vi "sendCmdFromTcpClientA.vi"(8 "error in (no error)":errorcluster, 11 "connectionID_A":refnum<k5>) -> (0 "error out":errorcluster, 2 "ack received":string[](array[string]), 3 "connectionID_A":refnum<k5>)   [LabVIEW 2018]
doc: "Generate commands as JSON packets and send them to TCP server, and then read the response from TCP server."
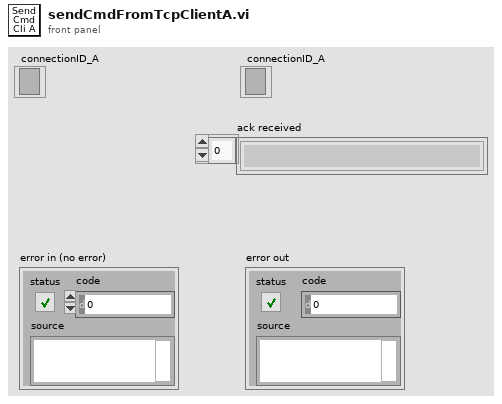
[diagram p1: front panel]
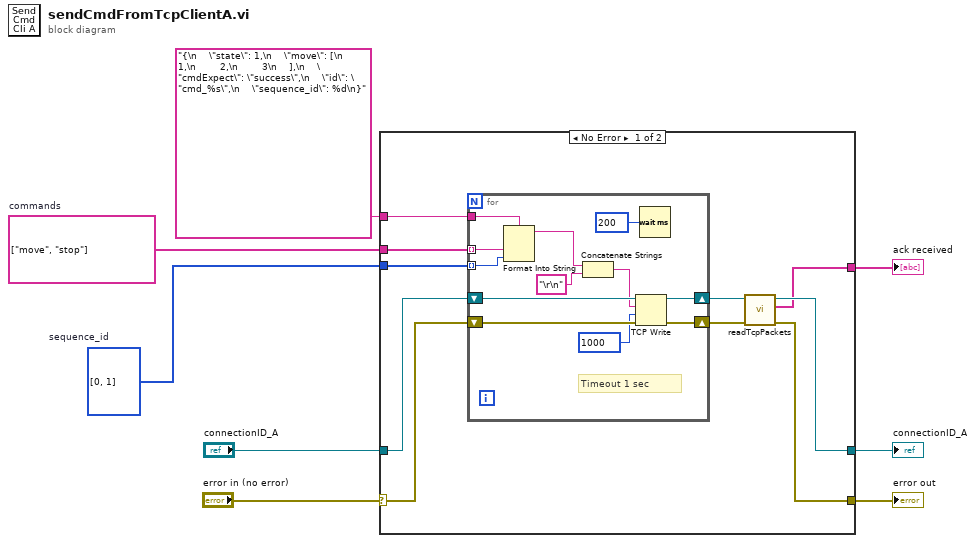
[diagram p0: block diagram]
diagram:
  w1 = i32[] [0, 1]  # sequence_id
  w2 = string[] ["move", "stop"]  # commands
  n1 = case shown="No Error" "error in (no error)" {
    selector: "error in (no error)" -> [w9 w32]
    tunnel: [w13 w31] -> w8
    tunnel: [w12 w32] -> w6
    tunnel: [w11 _] -> w5
    tunnel: "connectionID_A" -> [w18 w31]
    tunnel: "{\n    \"state\": 1,\n    \"move\": [\n        1,\n        2,\n        3\n    ],\n    \"cmdExpect\": \"success\",\n    \"id\": \"cmd_%s\",\n    \"sequence_id\": %d\n}" ("Display") -> [w10 _]
    tunnel: w2 -> [w17 _]
    tunnel: w1 -> [w16 _]
    frame No Error {
      n2 = for {
        shift-right: [w29] -> w14
        shift-left: w9 -> [w25]
        shift-right: [w27] -> w15
        shift-left: w18 -> [w26]
        tunnel: w10 -> [w23]
        tunnel: w17 -> [w22] mode=indexing
        tunnel: w16 -> [w21] mode=indexing
        # "Timeout 1 sec"
        n3 = Format Into String(format string=w23, w22, w21) -> (resulting string=w20:string)  [unwired: 2 in, 1 out]
        n4 = Concatenate Strings(w20, "\r\n" ("string")) -> (w24:string)
        n5 = TCP Write(connection ID=w26, data in=w24, error in (no error)=w25, 9:1000 ("timeout ms (25000)")) -> (connection ID out=w27:refnum<k5>, error out=w29:errorcluster)  [unwired: 1 out]
        n6 = Wait (ms)(milliseconds to wait=u32 200) -> ()  [unwired: 1 out]
      }
      n7 = call "readTcpPackets.vi"("error in (no error)"=w14, "connection ID in"=w15) -> ("error out"=w12:errorcluster, "TCP packets"=w11:string[], "connection ID out"=w13:refnum<k5>)  [unwired: 7 in]
    }
    frame Error {
    }
  }
  "connectionID_A" <- w8
  "error out" <- w6
  "ack received" <- w5
